vi "wRL to Q.vi"(1 "Wavelength":dbl format="%.4f", 2 "Radius of Curvature":dbl format="%.2f", 3 "beam radius(w)":dbl format="%.2f") -> (0 "Q":cdb format="%.2f")   [LabVIEW 2016]
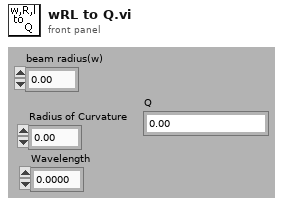
[diagram p1: front panel]
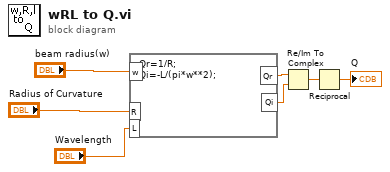
[diagram p0: block diagram]
diagram:
  n1 = formula code="Qr=1/R;\nQi=-L/(pi*w**2);"("w"="beam radius(w)", "R"="Radius of Curvature", "L"="Wavelength") -> ("Qr"=w4:dbl, "Qi"=w3:dbl)
  n2 = Re/Im To Complex(1:w3, 2:w4) -> (0:w2:cdb)
  n3 = Reciprocal(x=w2) -> (1/x=→"Q":cdb)
